vi "SampleRelativeMove.vi"() -> ()   [LabVIEW 2019]
panel:
  in  "Relative Steps":i32
  in  "Motor Number":i32=1
  in  "stop":bool
  out "Position Status":i32
  out "error out":errorcluster
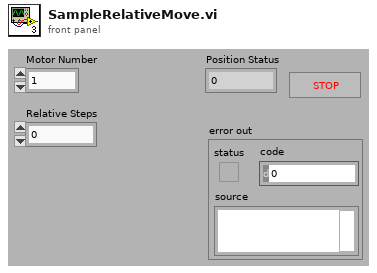
[diagram p1: front panel]
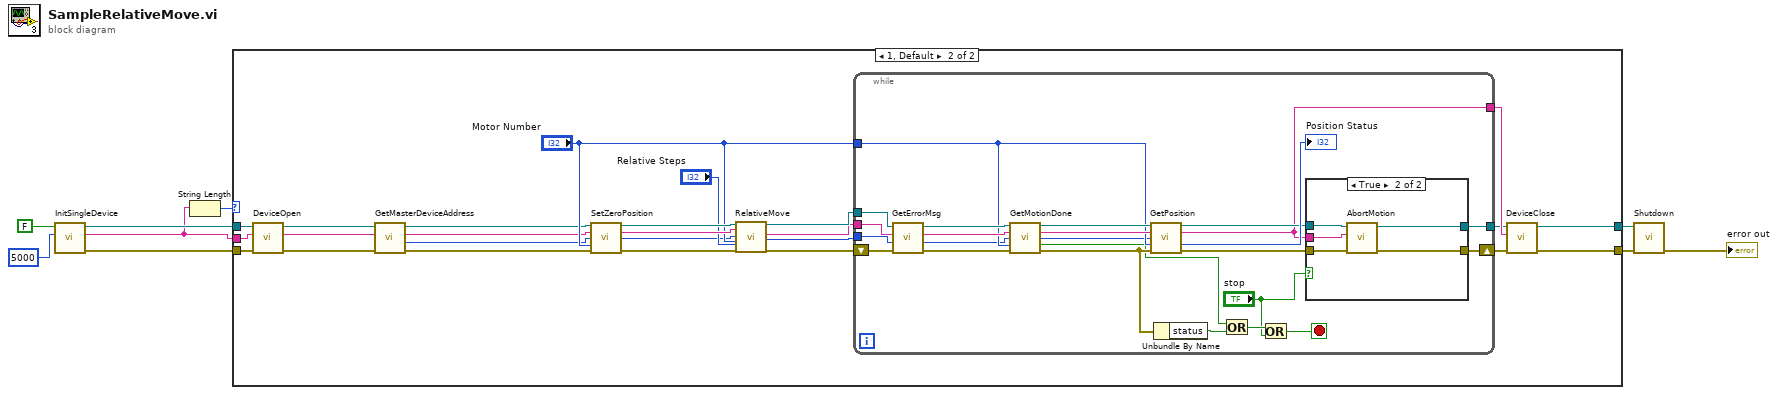
[diagram p0: block diagram]
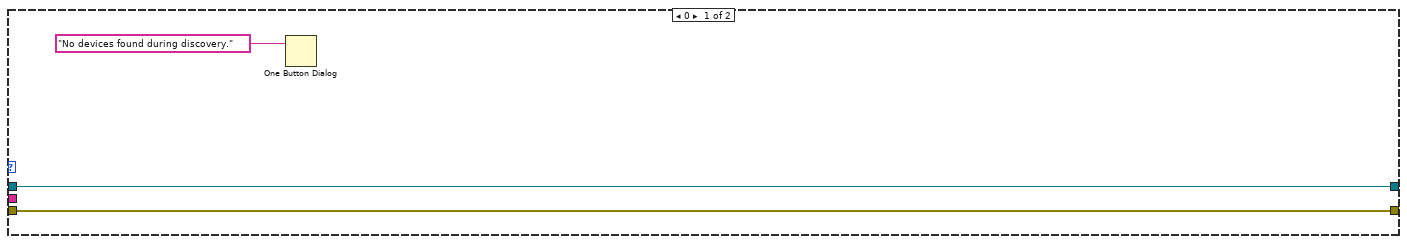
[diagram p2: hidden frame]
diagram:
  n1 = call "InitSingleDevice.vi"("msecDelayForDiscovery"=5000, "logging"=FALSE) -> ("error out"=w1:errorcluster, "DeviceKey Out"=w2:string, "CmdLib Out"=w4:refnum<k24>)  [unwired: 3 in]
  n2 = String Length(string=w2) -> (length=w3:i32)
  n3 = case shown="1, Default" w3 {
    tunnel: [w11 w13] -> w6
    tunnel: [w10 w15] -> w5
    tunnel: w4 -> [w11 w19]
    tunnel: w2 -> [_ w21]
    tunnel: w1 -> [w10 w23]
    frame 0 {
      n4 = One Button Dialog(message="No devices found during discovery.") -> ()  [unwired: 1 in, 1 out]
    }
    frame 1, Default {
      n5 = call "DeviceOpen.vi"("error in (no error)"=w23, "DeviceKey In"=w21, "CmdLib In"=w19) -> ("error out"=w22:errorcluster, "DeviceKey Out"=w20:string, "CmdLib Out"=w18:refnum<k24>)  [unwired: 2 in]
      n6 = call "GetMasterDeviceAddress.vi"("error in (no error)"=w22, "DeviceKey In"=w20, "CmdLib In"=w18) -> ("error out"=w28:errorcluster, "Device Address"=w29:i32, "DeviceKey Out"=w26:string, "CmdLib Out"=w27:refnum<k24>)  [unwired: 1 in]
      n7 = call "SetZeroPosition.vi"("CmdLib In"=w27, "DeviceKey In"=w26, "Device Address In"=w29, "Motor"="Motor Number", "error in (no error)"=w28) -> ("CmdLib Out"=w34:refnum<k24>, "DeviceKey Out"=w33:string, "Device Address Out"=w25:i32, "error out"=w32:errorcluster)  [unwired: 7 in]
      n8 = call "RelativeMove.vi"("CmdLib In"=w34, "DeviceKey In"=w33, "Device Address In"=w25, "Motor"="Motor Number", "Relative Steps"="Relative Steps", "error in (no error)"=w32) -> ("CmdLib Out"=w37:refnum<k24>, "DeviceKey Out"=w36:string, "Device Address Out"=w24:i32, "error out"=w35:errorcluster)  [unwired: 10 in]
      n9 = while {
        tunnel: "Motor Number" -> [w57]
        tunnel: w37 -> [w56]
        tunnel: w36 -> [w55]
        tunnel: [w42] -> w14
        tunnel: w24 -> [w41]
        shift-right: [w44] -> w16
        shift-left: w35 -> [w54]
        tunnel: [w38] -> w17
        stop <- w47 stop-if-true
        n10 = call "GetErrorMsg.vi"("error in (no error)"=w54, "Device Address In"=w41, "DeviceKey In"=w55, "CmdLib In"=w56) -> ("error out"=w53:errorcluster, "Device Address Out"=w40:i32, "DeviceKey Out"=w59:string, "CmdLib Out"=w58:refnum<k24>)
        n11 = call "GetMotionDone.vi"("CmdLib In"=w58, "DeviceKey In"=w59, "Device Address In"=w40, "Motor"=w57, "error in (no error)"=w53) -> ("CmdLib Out"=w60:refnum<k24>, "DeviceKey Out"=w61:string, "Device Address Out"=w39:i32, "Is Motion Done"=w50:bool, "error out"=w51:errorcluster)  [unwired: 6 in]
        n12 = call "GetPosition.vi"("CmdLib In"=w60, "DeviceKey In"=w61, "Device Address In"=w39, "Motor"=w57, "error in (no error)"=w51) -> ("CmdLib Out"=w43:refnum<k24>, "DeviceKey Out"=w38:string, "Position"=→"Position Status":i32, "error out"=w45:errorcluster)  [unwired: 6 in, 1 out]
        n13 = Unbundle By Name(w51) -> ("status"=w52:bool)
        n14 = Or(x=w50, y=w52) -> (x .or. y?=w48:bool)
        n15 = Or(x=w48, y="stop") -> (x .or. y?=w47:bool)
        n16 = case shown="True" "stop" {
          tunnel: w45 -> [w62 w68]
          tunnel: [w62 w67] -> w44
          tunnel: w43 -> [w63 w66]
          tunnel: [w63 w65] -> w42
          tunnel: w38 -> [_ w64]
          frame False {
          }
          frame True {
            n17 = call "AbortMotion.vi"("error in (no error)"=w68, "DeviceKey In"=w64, "CmdLib In"=w66) -> ("error out"=w67:errorcluster, "CmdLib Out"=w65:refnum<k24>)  [unwired: 1 in, 2 out]
          }
        }
      }
      n18 = call "DeviceClose.vi"("error in (no error)"=w16, "DeviceKey In"=w17, "CmdLib In"=w14) -> ("error out"=w15:errorcluster, "CmdLib Out"=w13:refnum<k24>)  [unwired: 2 in, 1 out]
    }
  }
  n19 = call "Shutdown.vi"("error in (no error)"=w5, "CmdLib In"=w6) -> ("error out"=→"error out":errorcluster)  [unwired: 4 in, 1 out]
